vi "FTW-JSON-MergeObject.vi"(8 "error in (no error)":errorcluster, 9 "Initial JSON String (\"\")":string, 10 "Cluster to Merge":variant, 11 "Update Mode (0: Upsert)":T1) -> (0 "error out":errorcluster, 3 "Merged JSON String (UTF-8)":string)   [LabVIEW 2015]
doc: "This VI merges two JSON strings together."
uses:
  FTW-JSON-JoinMode.ctl
  container/FTW-Container.lvclass
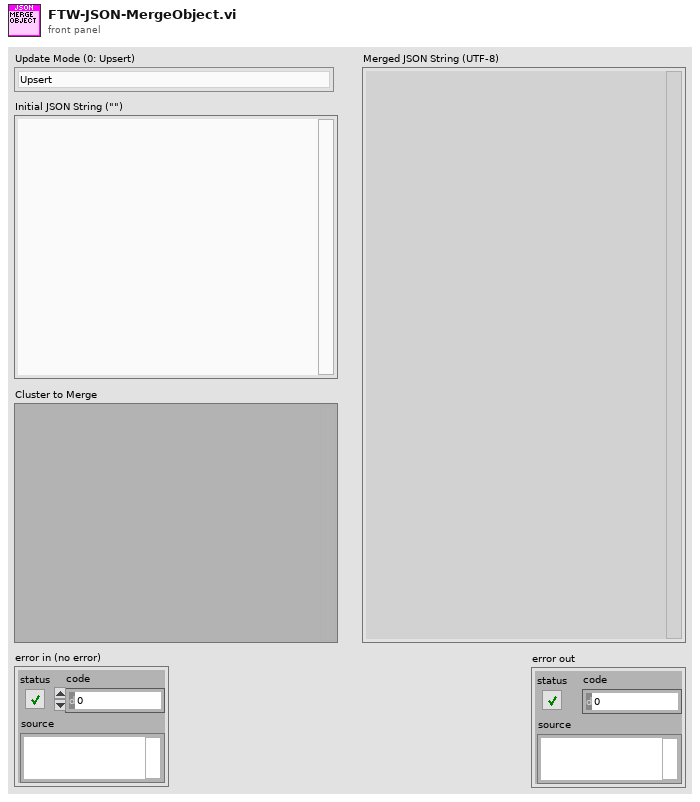
[diagram p1: front panel]
types:
  T1 = typedef "FTW-JSON-JoinMode.ctl" = enum32{"Upsert", "Update Only", "Insert Only"}
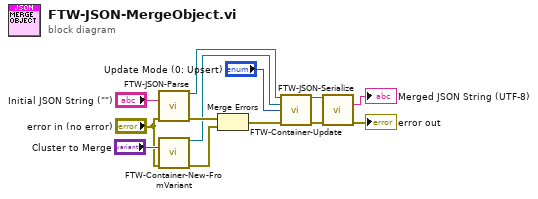
[diagram p0: block diagram]
diagram:
  n1 = call "FTW-JSON-Parse.vi"("JSON String"="Initial JSON String (\"\")", "error in"="error in (no error)") -> ("Container"=w6:refnum<class "FTW-Container.lvclass">, "error out"=w5:errorcluster)  [unwired: 12 in]
  n2 = call "FTW-Container-New-FromVariant.vi"("Variant"="Cluster to Merge", "error in"="error in (no error)") -> ("FTW-Container"=w2:refnum<class "FTW-Container.lvclass">, "error out"=w4:errorcluster)  [unwired: 12 in]
  n3 = Merge Errors(w5, w4) -> (w10:errorcluster)
  n4 = call "FTW-Container-Update.vi"("FTW-Container In"=w6, "Other Container"=w2, "Join Mode"="Update Mode (0: Upsert)", "error in"=w10) -> ("Updated Container"=w7:refnum<class "FTW-Container.lvclass">, "error out"=w8:errorcluster)  [unwired: 10 in]
  n5 = call "FTW-JSON-Serialize.vi"("JSON"=w7, "error in"=w8) -> ("JSON String (UTF-8)"=→"Merged JSON String (UTF-8)":string, "error out"=→"error out":errorcluster)  [unwired: 11 in, 1 out]
